vi "A basic actor.vi"() -> ()   [LabVIEW 2013]
uses:
  <vilib>/DAQmx/read.llb/DAQmx Read (Analog 1D DBL 1Chan NSamp).vi
panel:
  in  "Start":bool
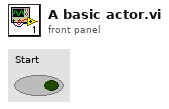
[diagram p1: front panel]
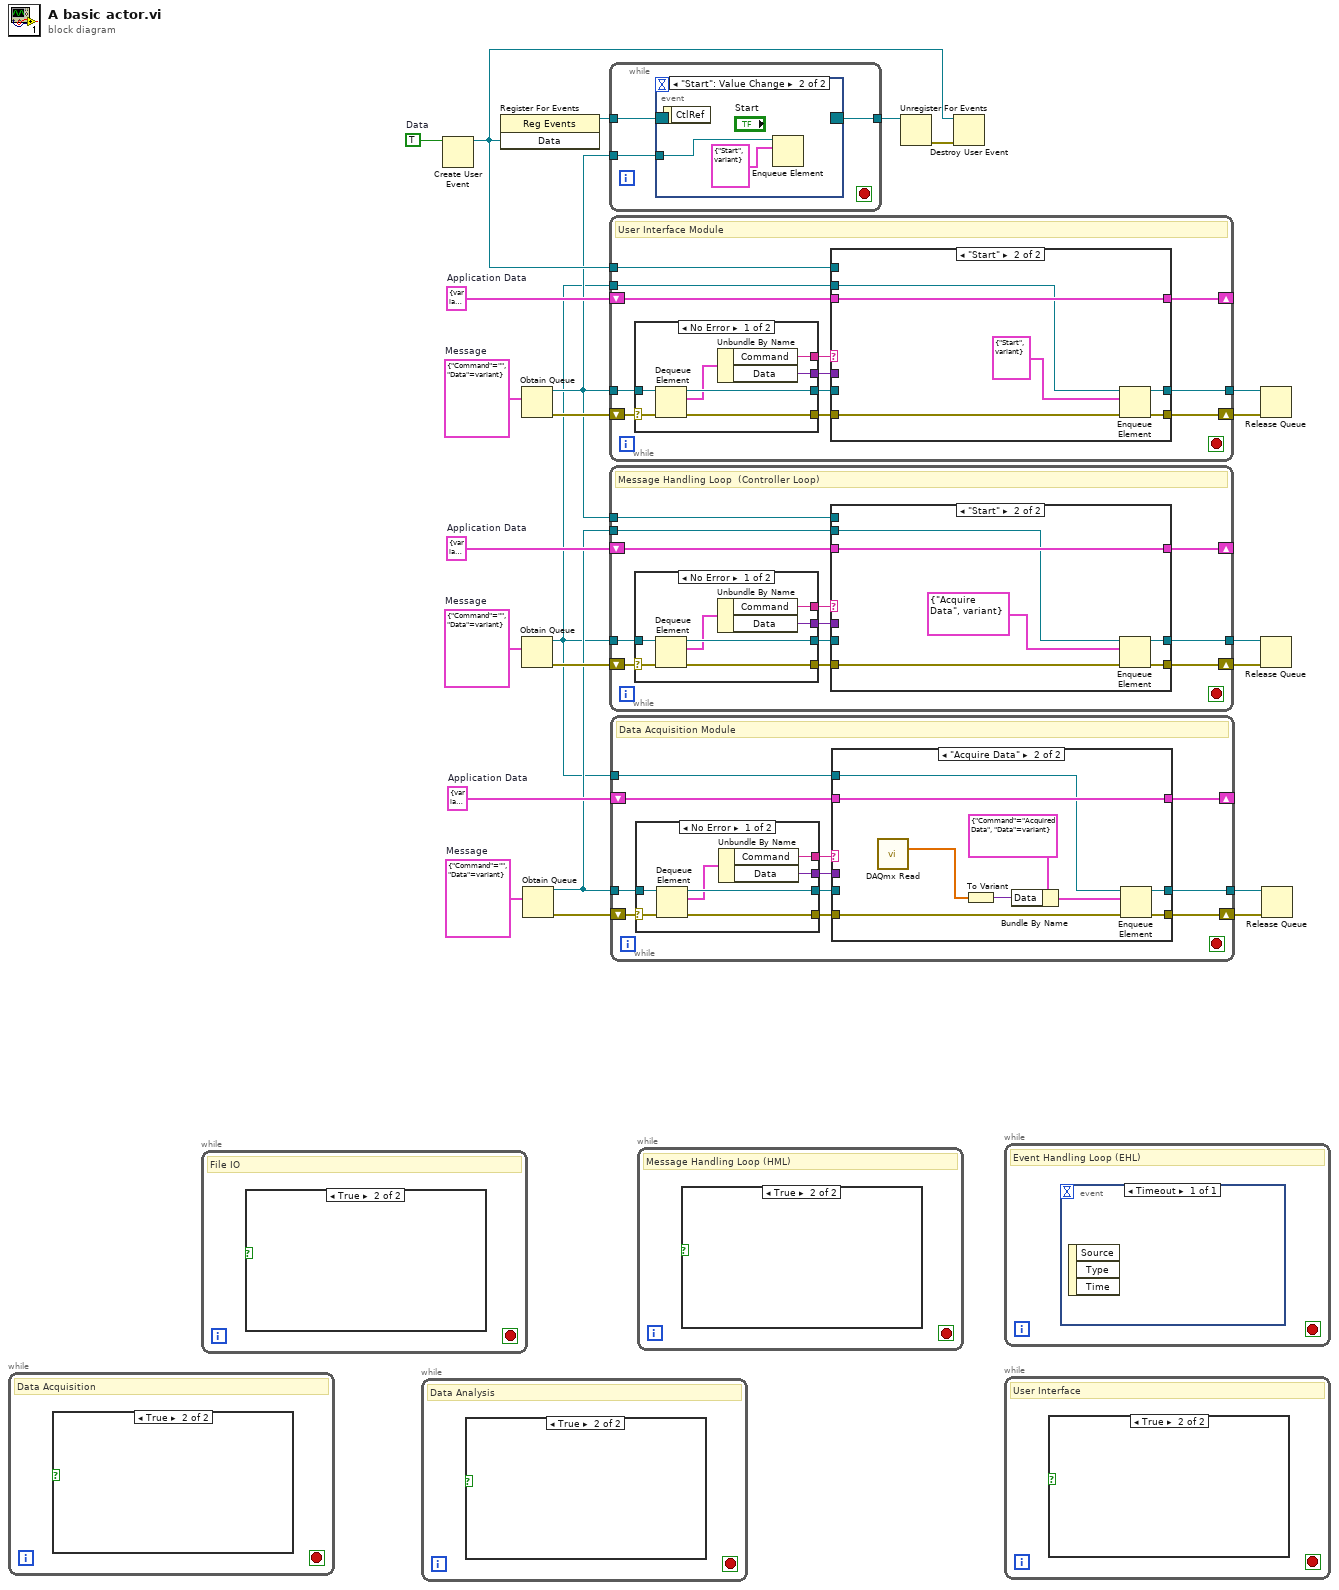
[diagram p0: block diagram]
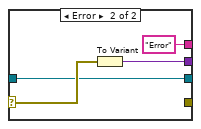
[diagram p2: hidden frame]
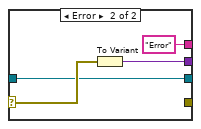
[diagram p4: hidden frame]
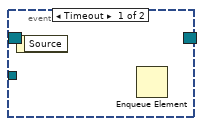
[diagram p11: hidden frame]
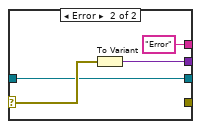
[diagram p12: hidden frame]
diagram:
  w5 = cluster{variant} {variant}  # Application Data
  w6 = cluster{"Command":string, "Data":variant} {"Command"="", "Data"=variant}  # Message
  w14 = cluster{variant} {variant}  # Application Data
  w13 = cluster{"Command":string, "Data":variant} {"Command"="", "Data"=variant}  # Message
  w17 = TRUE  # Data
  w19 = cluster{variant} {variant}  # Application Data
  w20 = cluster{"Command":string, "Data":variant} {"Command"="", "Data"=variant}  # Message
  n1 = while {
    stop <- _ stop-if-true
    # "Data Acquisition"
    n2 = case shown="True" {
      selector: _ -> [_ _]
      frame False {
      }
      frame True {
      }
    }
  }
  n3 = while {
    stop <- _ stop-if-true
    # "File IO"
    n4 = case shown="True" {
      selector: _ -> [_ _]
      frame False {
      }
      frame True {
      }
    }
  }
  n5 = while {
    stop <- _ stop-if-true
    # "Data Analysis"
    n6 = case shown="True" {
      selector: _ -> [_ _]
      frame False {
      }
      frame True {
      }
    }
  }
  n7 = Create User Event(user event datatype=w17) -> (user event=w4:refnum<user-event>)  [unwired: 1 in, 1 out]
  n8 = register-events(w4) -> (reference out=w16:refnum<event-registration>)  [unwired: 2 in, 1 out]
  n9 = Obtain Queue(element data type=w6) -> (queue out=w2:refnum<queue>, error out=w9:errorcluster)  [unwired: 4 in, 1 out]
  n10 = Obtain Queue(element data type=w13) -> (queue out=w1:refnum<queue>, error out=w10:errorcluster)  [unwired: 4 in, 1 out]
  n11 = Obtain Queue(element data type=w20) -> (queue out=w3:refnum<queue>, error out=w23:errorcluster)  [unwired: 4 in, 1 out]
  n12 = while {
    tunnel: [w26] -> w18
    tunnel: w16 -> [w25]
    tunnel: w2 -> [w24]
    stop <- _ stop-if-true
    n13 = event shown="[1] \"Start\": Value Change" {
      selector: w25 -> [_ _]
      dyn-events: [_ _] -> w26
      timeout: _ -> [_ _]
      tunnel: w24 -> [_ w28]
      event Timeout {
        n14 = event-data() -> ()  [unwired: 1 in, 1 out]
        n15 = Enqueue Element() -> ()  [unwired: 4 in, 3 out]
      }
      event "Start": Value Change {
        n16 = event-data() -> ()  [unwired: 1 in, 1 out]
        n17 = Enqueue Element(queue=w28, element=cluster{"Command":string, "Data":variant} {"Command"="Start", "Data"=variant}) -> ()  [unwired: 2 in, 3 out]
      }
    }
  }
  n18 = while {
    tunnel: w2 -> [w40]
    tunnel: [w36] -> w8
    shift-right: [w34] -> _
    shift-left: w5 -> [w33]
    shift-right: [w35] -> w7
    shift-left: w9 -> [w39]
    tunnel: w4 -> [w30]
    tunnel: w1 -> [w29]
    stop <- _ stop-if-true
    # "User Interface Module"
    n19 = case shown="No Error" w39 {
      selector: w39 -> [w46 w51]
      tunnel: w40 -> [w47 w48]
      tunnel: [w45 w48] -> w38
      tunnel: [w44 _] -> w37
      tunnel: [w42 "Error" ("Command")] -> w32
      tunnel: [w41 w50] -> w31
      frame No Error {
        n20 = Dequeue Element(queue=w47, error in (no error)=w46) -> (queue out=w45:refnum<queue>, element=w43:cluster{"Command":string, "Data":variant}, error out=w44:errorcluster)  [unwired: 1 in, 1 out]
        n21 = Unbundle By Name(w43) -> ("Command"=w42:string, "Data"=w41:variant)
      }
      frame Error {
        n22 = To Variant(anything=w51) -> (Variant=w50:variant)
      }
    }
    n23 = case shown="\"Start\"" w32 {
      tunnel: w38 -> [w53 _]
      tunnel: w37 -> [w52 w60]
      tunnel: [w53 w59] -> w36
      tunnel: [w52 w58] -> w35
      tunnel: [w54 w57] -> w34
      tunnel: w33 -> [w54 w57]
      tunnel: w31 -> [_ _]
      tunnel: w30 -> [_ _]
      tunnel: w29 -> [_ w55]
      frame "False", Default {
      }
      frame "Start" {
        n24 = Enqueue Element(queue=w55, element=cluster{"Command":string, "Data":variant} {"Command"="Start", "Data"=variant}, error in (no error)=w60) -> (queue out=w59:refnum<queue>, error out=w58:errorcluster)  [unwired: 1 in, 1 out]
      }
    }
  }
  n25 = while {
    tunnel: w1 -> [w72]
    tunnel: [w68] -> w11
    shift-right: [w66] -> _
    shift-left: w14 -> [w65]
    shift-right: [w67] -> w12
    shift-left: w10 -> [w71]
    tunnel: w2 -> [w62]
    tunnel: w3 -> [w61]
    stop <- _ stop-if-true
    # "Message Handling Loop  (Controller Loop)"
    n26 = case shown="No Error" w71 {
      selector: w71 -> [w78 w83]
      tunnel: w72 -> [w79 w80]
      tunnel: [w77 w80] -> w70
      tunnel: [w76 _] -> w69
      tunnel: [w74 "Error" ("Command")] -> w64
      tunnel: [w73 w82] -> w63
      frame No Error {
        n27 = Dequeue Element(queue=w79, error in (no error)=w78) -> (queue out=w77:refnum<queue>, element=w75:cluster{"Command":string, "Data":variant}, error out=w76:errorcluster)  [unwired: 1 in, 1 out]
        n28 = Unbundle By Name(w75) -> ("Command"=w74:string, "Data"=w73:variant)
      }
      frame Error {
        n29 = To Variant(anything=w83) -> (Variant=w82:variant)
      }
    }
    n30 = case shown="\"Start\"" w64 {
      tunnel: w70 -> [w85 _]
      tunnel: w69 -> [w84 w92]
      tunnel: [w85 w91] -> w68
      tunnel: [w84 w90] -> w67
      tunnel: [w86 w89] -> w66
      tunnel: w65 -> [w86 w89]
      tunnel: w63 -> [_ _]
      tunnel: w62 -> [_ _]
      tunnel: w61 -> [_ w88]
      frame "False", Default {
      }
      frame "Start" {
        n31 = Enqueue Element(queue=w88, element=cluster{"Command":string, "Data":variant} {"Command"="Acquire Data", "Data"=variant}, error in (no error)=w92) -> (queue out=w91:refnum<queue>, error out=w90:errorcluster)  [unwired: 1 in, 1 out]
      }
    }
  }
  n32 = while {
    tunnel: w3 -> [w103]
    tunnel: [w99] -> w22
    shift-right: [w97] -> _
    shift-left: w19 -> [w96]
    shift-right: [w98] -> w21
    shift-left: w23 -> [w102]
    tunnel: w1 -> [w93]
    stop <- _ stop-if-true
    # "Data Acquisition Module"
    n33 = case shown="No Error" w102 {
      selector: w102 -> [w109 w114]
      tunnel: w103 -> [w110 w111]
      tunnel: [w108 w111] -> w101
      tunnel: [w107 _] -> w100
      tunnel: [w105 "Error" ("Command")] -> w95
      tunnel: [w104 w113] -> w94
      frame No Error {
        n34 = Dequeue Element(queue=w110, error in (no error)=w109) -> (queue out=w108:refnum<queue>, element=w106:cluster{"Command":string, "Data":variant}, error out=w107:errorcluster)  [unwired: 1 in, 1 out]
        n35 = Unbundle By Name(w106) -> ("Command"=w105:string, "Data"=w104:variant)
      }
      frame Error {
        n36 = To Variant(anything=w114) -> (Variant=w113:variant)
      }
    }
    n37 = case shown="\"Acquire Data\"" w95 {
      tunnel: w101 -> [w116 _]
      tunnel: w100 -> [w115 w126]
      tunnel: [w116 w125] -> w99
      tunnel: [w115 w124] -> w98
      tunnel: [w117 w123] -> w97
      tunnel: w96 -> [w117 w123]
      tunnel: w94 -> [_ _]
      tunnel: w93 -> [_ w122]
      frame "False", Default {
      }
      frame "Acquire Data" {
        n38 = call-poly <vilib>:"DAQmx Read.vi"() -> ("data"=w118:dbl[])  [unwired: 13 in, 2 out]
        n39 = To Variant(anything=w118) -> (Variant=w119:variant)
        n40 = Bundle By Name(cluster=cluster{"Command":string, "Data":variant} {"Command"="Acquired Data", "Data"=variant} ("element"), "Data"=w119) -> (w120:cluster{"Command":string, "Data":variant})
        n41 = Enqueue Element(queue=w122, element=w120, error in (no error)=w126) -> (queue out=w125:refnum<queue>, error out=w124:errorcluster)  [unwired: 1 in, 1 out]
      }
    }
  }
  n42 = while {
    stop <- _ stop-if-true
    # "Message Handling Loop (HML)"
    n43 = case shown="True" {
      selector: _ -> [_ _]
      frame False {
      }
      frame True {
      }
    }
  }
  n44 = Unregister For Events(event registration refnum=w18) -> (error out=w15:errorcluster)  [unwired: 1 in]
  n45 = Destroy User Event(user event=w4, error in=w15) -> ()  [unwired: 1 out]
  n46 = while {
    stop <- _ stop-if-true
    # "Event Handling Loop (EHL)"
    n47 = event shown="[0] Timeout" {
      selector: _ -> [_]
      dyn-events: _ -> [_]
      timeout: _ -> [_]
      event Timeout {
        n48 = event-data() -> ()  [unwired: 1 in, 3 out]
      }
    }
  }
  n49 = while {
    stop <- _ stop-if-true
    # "User Interface"
    n50 = case shown="True" {
      selector: _ -> [_ _]
      frame False {
      }
      frame True {
      }
    }
  }
  n51 = Release Queue(queue=w8, error in (no error)=w7) -> ()  [unwired: 1 in, 3 out]
  n52 = Release Queue(queue=w11, error in (no error)=w12) -> ()  [unwired: 1 in, 3 out]
  n53 = Release Queue(queue=w22, error in (no error)=w21) -> ()  [unwired: 1 in, 3 out]
